vi "moveby_single_channel.vi"(4 "Desired Position":dbl) -> (1 "Sensor Sampling":waveform(dbl)[](graph), 2 "Absolute vs. Desired Pos.":cluster{dbl, "Position":dbl}(graph) caption="Waveform Chart")   [LabVIEW 2020]
uses:
  C:/Users/359167/Documents/LabVIEW_ws/Thorlabs.MotionControl.DeviceManagerCLI.dll
  Thorlabs.MotionControl.DeviceManagerCLI.dll
  C:/Users/359167/Documents/LabVIEW_ws/Thorlabs.MotionControl.KCube.InertialMotorCLI.dll
  Thorlabs.MotionControl.KCube.InertialMotorCLI.dll
  <vilib>/DAQmx/read.llb/DAQmx Read (Analog 1D Wfm NChan NSamp).vi
  <vilib>/Analysis/baseanly.llb/Mean (DBL).vi
  <vilib>/DAQmx/create/channels.llb/DAQmx Create Channel (AI-Voltage-Basic).vi
  <vilib>/DAQmx/configure/timing.llb/DAQmx Timing (Sample Clock).vi
  <vilib>/Utility/file.llb/Read Delimited Spreadsheet (DBL).vi
  <vilib>/DAQmx/miscellaneous.llb/DAQmx Fill In Error Info.vi
  <vilib>/Utility/file.llb/Write Delimited Spreadsheet (DBL).vi
  <vilib>/Analysis/NI_AALBase.lvlib
panel:
  in  "Path 2":path=path "C:/Users/359167/Documents/saved.csv"
  in  "Path":path=path "C:/Users/359167/Documents/saved.csv"
  out "Saved File Data":dbl[][](array[numeric])
  out "Absolute Pos.":dbl
  out "degree error":dbl format="%#.3f"
  out "Step Size":i32
  out "Relative Pos.":dbl
  # "Channel"
  # "Saved Abs. Pos."
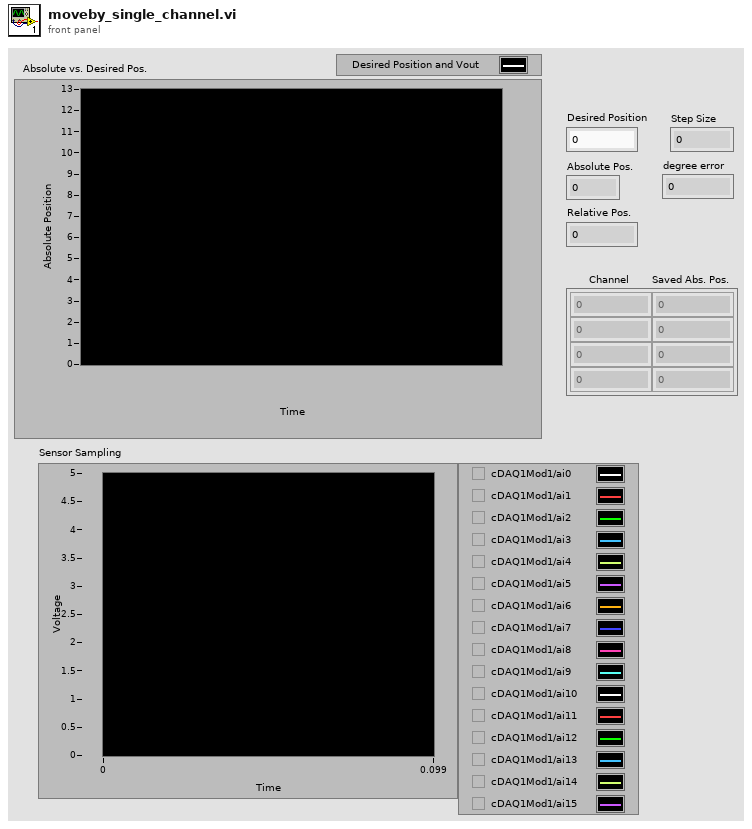
[diagram p1: front panel]
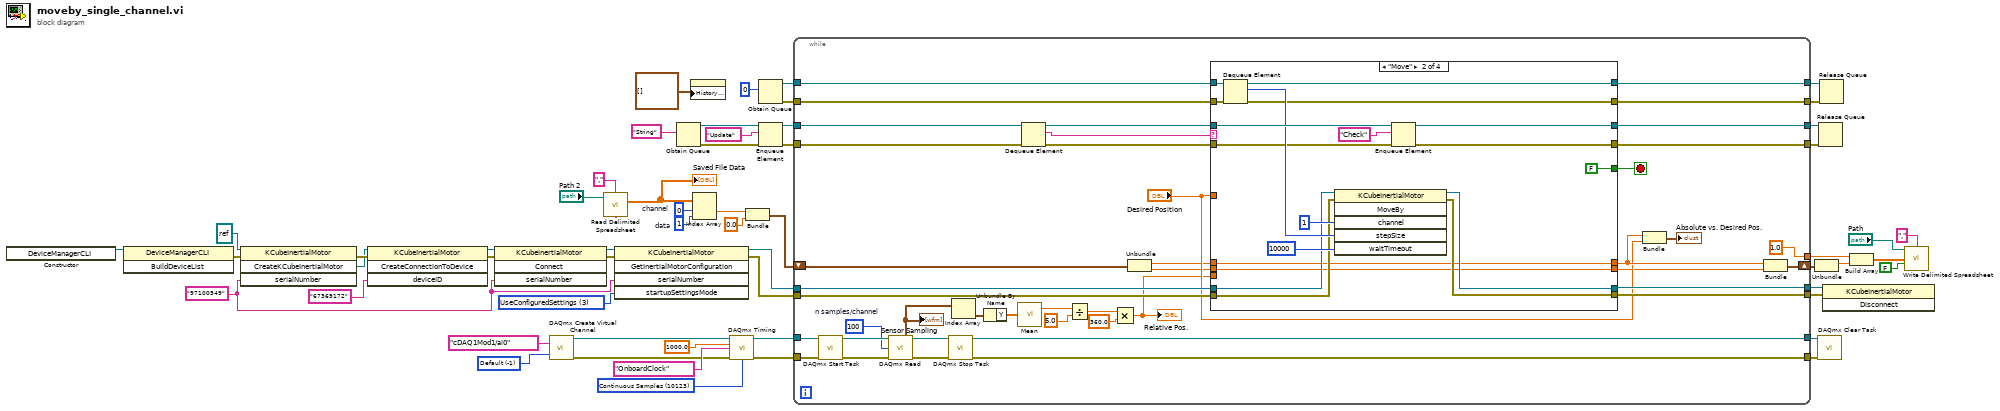
[diagram p0: block diagram]
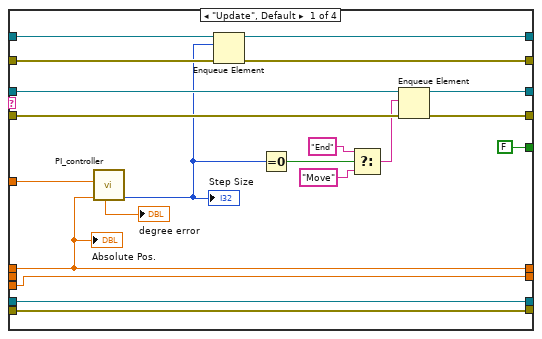
[diagram p2: hidden frame]
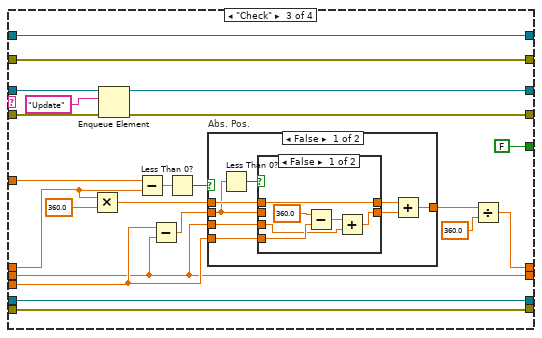
[diagram p3: hidden frame]
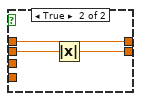
[diagram p4: hidden frame]
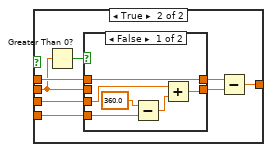
[diagram p5: hidden frame]
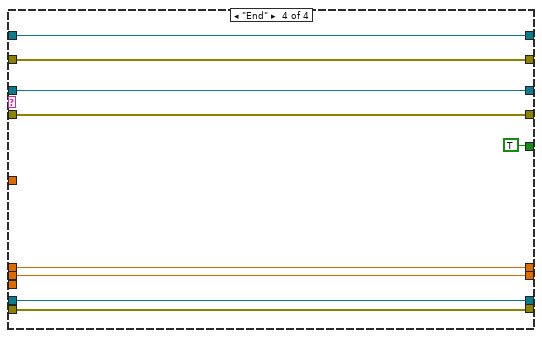
[diagram p7: hidden frame]
diagram:
  w8 = 3 items=["UseDeviceSettings"=1, "UseFileSettings"=2, "UseConfiguredSettings"=3] ("startupSettingsMode")
  w13 = "97100549" ("SerialNumber")
  w34 = -1 items=["Default"=-1, "RSE"=10083, "NRSE"=10078, "Differential"=10106, "Pseudodifferential"=12529] ("input terminal configuration")
  w35 = 10123 items=["Finite Samples"=10178, "Continuous Samples"=10123, "Hardware Timed Single Point"=12522] ("sample mode")
  w36 = 1  # data
  w37 = 0  # channel
  n1 = constructor class="DeviceManagerCLI"() -> (reference out=w26:refnum<k24>)  [unwired: 3 in, 2 out]
  n2 = invoke class="DeviceManagerCLI" method="BuildDeviceList"(reference=w26) -> (error out=w24:errorcluster)  [unwired: 2 in, 2 out]
  n3 = invoke class="KCubeInertialMotor" method="CreateKCubeInertialMotor"(reference=refnum<k24> refnum, error in=w24, "serialNumber"=w13) -> (error out=w23:errorcluster, "CreateKCubeInertialMotor"=w22:refnum<k24>)  [unwired: 1 in, 2 out]
  n4 = invoke class="KCubeInertialMotor" method="CreateConnectionToDevice"(reference=w22, error in=w23, "deviceID"="67369172") -> (reference out=w10:refnum<k24>, error out=w9:errorcluster)  [unwired: 1 in, 2 out]
  n5 = invoke class="KCubeInertialMotor" method="Connect"(reference=w10, error in=w9, "serialNumber"=w13) -> (reference out=w12:refnum<k24>, error out=w11:errorcluster)  [unwired: 1 in, 2 out]
  n6 = call-poly <vilib>:"DAQmx Create Virtual Channel.vi"("input terminal configuration"=w34, "physical channels"=tag "cDAQ1Mod1/ai0" ("DAQmx Physical Channel")) -> ("task out"=w30:refnum<k21>, "error out"=w31:errorcluster)  [unwired: 12 in]
  n7 = call-poly <vilib>:"Read Delimited Spreadsheet.vi"("file path (dialog if empty)"="Path 2", "delimiter (\\t)"="," ("delimiter (\\t)")) -> ("all rows"=w38:dbl[][])  [unwired: 8 in, 5 out]
  "Saved File Data" <- w38
  n8 = invoke class="KCubeInertialMotor" method="GetInertialMotorConfiguration"(reference=w12, error in=w11, "serialNumber"=w13, "startupSettingsMode"=w8) -> (reference out=w7:refnum<k24>, error out=w6:errorcluster)  [unwired: 1 in, 3 out]
  n9 = Obtain Queue(element data type="String") -> (queue out=w43:refnum<queue>, error out=w42:errorcluster)  [unwired: 4 in, 1 out]
  n10 = property on="Absolute vs. Desired Pos." class="WFChart (strict)"("History Data"=cluster{dbl, "Position":dbl}[] []) -> ()  [unwired: 2 in, 2 out]
  n11 = Index Array(array=w38, index (row)=w37, index (col)=w36) -> (element=w3:dbl)
  n12 = call-poly <vilib>:"DAQmx Timing.vi"("task/channels in"=w30, "sample mode"=w35, "rate"=1000.0 ("sample rate"), "source"=tag "OnboardClock", "error in"=w31) -> ("task out"=w29:refnum<k21>, "error out"=w28:errorcluster)  [unwired: 9 in]
  n13 = Bundle("Numeric"=w3, 0.0) -> (w2:cluster{"Numeric":dbl, dbl})  [unwired: 1 in]
  n14 = Obtain Queue(element data type=0) -> (queue out=w50:refnum<queue>, error out=w49:errorcluster)  [unwired: 4 in, 1 out]
  n15 = Enqueue Element(queue=w43, element="Update", error in (no error)=w42) -> (queue out=w41:refnum<queue>, error out=w40:errorcluster)  [unwired: 1 in, 1 out]
  n16 = while {
    tunnel: w50 -> [w86]
    tunnel: [w89] -> w52
    tunnel: [w90] -> w51
    tunnel: w49 -> [w88]
    tunnel: w40 -> [w71]
    tunnel: [w87] -> w48
    tunnel: [w74] -> w47
    tunnel: [w68] -> w46
    tunnel: [w67] -> w45
    tunnel: w41 -> [w72]
    tunnel: [1.0] -> w18
    tunnel: w7 -> [w65]
    tunnel: w6 -> [w64]
    tunnel: w29 -> [w94]
    tunnel: [w92] -> w56
    tunnel: w28 -> [w93]
    tunnel: [w91] -> w55
    shift-right: [w66] -> w5
    shift-left: w2 -> [w60]
    stop <- w96 stop-if-true
    w81 = 100  # n samples/channel
    # "Consumer"
    n17 = call <vilib>:"DAQmx Start Task.vi"("task/channels in"=w94, "error in"=w93) -> ("task out"=w82:refnum<k21>, "error out"=w83:errorcluster)  [unwired: 12 in]
    n18 = call-poly <vilib>:"DAQmx Read.vi"("task/channels in"=w82, "number of samples per channel"=w81, "error in"=w83) -> ("data"=w70:waveform(dbl)[], "task out"=w84:refnum<k21>, "error out"=w85:errorcluster)  [unwired: 10 in]
    "Sensor Sampling" <- w70
    n19 = call <vilib>:"DAQmx Stop Task.vi"("task/channels in"=w84, "error in"=w85) -> ("task out"=w92:refnum<k21>, "error out"=w91:errorcluster)  [unwired: 12 in]
    n20 = Index Array(array=w70) -> (element=w80:waveform(dbl))  [unwired: 1 in]
    n21 = Unbundle By Name(w80) -> ("Y"=w78:dbl[])
    n22 = call-poly <vilib>:"Mean.vi"("X"=w78) -> ("mean"=w77:dbl)  [unwired: 1 out]
    n23 = Dequeue Element(queue=w72, error in (no error)=w71) -> (queue out=w98:refnum<queue>, element=w97:string, error out=w95:errorcluster)  [unwired: 1 in, 1 out]
    n24 = Divide(x=w77, y=5.0) -> (x/y=w79:dbl)
    n25 = Multiply(x=w79, y=360.0) -> (x*y=w61:dbl)
    "Relative Pos." <- w61
    n26 = Unbundle(w60) -> ("Numeric"=w57:dbl, w58:dbl)
    n27 = case shown="\"Move\"" w97 {
      tunnel: w98 -> [w112 w135 w156 w198]
      tunnel: [w118 w125 w157 w199] -> w87
      tunnel: [FALSE FALSE FALSE TRUE] -> w96
      tunnel: w95 -> [w117 w132 w155 w199]
      tunnel: w86 -> [w116 w129 w154 w200]
      tunnel: w88 -> [w115 w131 w153 w197]
      tunnel: [w114 w128 w154 w200] -> w74
      tunnel: [w113 w130 w153 w197] -> w68
      tunnel: [w102 w137 w142 w195] -> w90
      tunnel: [w103 w136 w143 w196] -> w89
      tunnel: [w108 w127 w158 w198] -> w67
      tunnel: [w100 w120 w148 w194] -> w63
      tunnel: [w99 w119 w138 w193] -> w59
      tunnel: w65 -> [w102 w122 w142 w195]
      tunnel: w64 -> [w103 w121 w143 w196]
      tunnel: "Desired Position" -> [w101 _ w141 _]
      tunnel: w61 -> [w99 _ w140 _]
      tunnel: w57 -> [w100 w120 w139 w194]
      tunnel: w58 -> [_ w119 w138 w193]
      frame "Update", Default {
        n28 = call "PI_controller.vi"("absolute position"=w100, "desired position"=w101) -> ("step size"=w107:i32, "degree error"=→"degree error":dbl)  [unwired: 7 in, 1 out]
        "Step Size" <- w107
        n29 = Enqueue Element(queue=w116, element=w107, error in (no error)=w115) -> (queue out=w114:refnum<queue>, error out=w113:errorcluster)  [unwired: 1 in, 1 out]
        n30 = Equal To 0?(x=w107) -> (x = 0?=w105:bool)
        n31 = Select(t="End", s=w105, f="Move" ("element")) -> (s? t:f=w109:string)
        n32 = Enqueue Element(queue=w112, element=w109, error in (no error)=w117) -> (queue out=w108:refnum<queue>, error out=w118:errorcluster)  [unwired: 1 in, 1 out]
        "Absolute Pos." <- w100
      }
      frame "Move" {
        n33 = Dequeue Element(queue=w129, error in (no error)=w131) -> (queue out=w128:refnum<queue>, element=w134:i32, error out=w130:errorcluster)  [unwired: 1 in, 1 out]
        n34 = invoke class="KCubeInertialMotor" method="MoveBy"(reference=w122, error in=w121, "channel"=1 ("Channel"), "stepSize"=w134, "waitTimeout"=10000) -> (reference out=w137:refnum<k24>, error out=w136:errorcluster)  [unwired: 1 in, 4 out]
        n35 = Enqueue Element(queue=w135, element="Check", error in (no error)=w132) -> (queue out=w127:refnum<queue>, error out=w125:errorcluster)  [unwired: 1 in, 1 out]
      }
      frame "Check" {
        n36 = Multiply(x=w139, y=360.0) -> (x*y=w144:dbl)
        n37 = Enqueue Element(queue=w156, element="Update", error in (no error)=w155) -> (queue out=w158:refnum<queue>, error out=w157:errorcluster)  [unwired: 1 in, 1 out]
        n38 = Subtract(x=w141, y=w139) -> (x-y=w147:dbl)
        n39 = Subtract(x=w140, y=w138) -> (x-y=w146:dbl)
        n40 = Less Than 0?(x=w147) -> (x < 0?=w151:bool)
        n41 = case "Abs. Pos." shown="False" w151 {
          tunnel: w144 -> [w164 w184]
          tunnel: w138 -> [w166 w182]
          tunnel: [w165 w180] -> w150
          tunnel: w140 -> [w161 w178]
          tunnel: w146 -> [w160 w177]
          frame False {
            n42 = Less Than 0?(x=w160) -> (x < 0?=w167:bool)
            n43 = case shown="False" w167 {
              tunnel: w164 -> [w171 w176]
              tunnel: [w172 w174] -> w162
              tunnel: w166 -> [w168 _]
              tunnel: w161 -> [w169 _]
              tunnel: [w171 w176] -> w163
              tunnel: w160 -> [_ w175]
              frame False {
                n44 = Subtract(x=360.0 ("y"), y=w169) -> (x-y=w173:dbl)
                n45 = Add(x=w173, y=w168) -> (x+y=w172:dbl)
              }
              frame True {
                n46 = Absolute Value(x=w175) -> (abs(x)=w174:dbl)
              }
            }
            n47 = Add(x=w163, y=w162) -> (x+y=w165:dbl)
          }
          frame True {
            n48 = Greater Than 0?(x=w177) -> (x > 0?=w183:bool)
            n49 = case shown="False" w183 {
              tunnel: w184 -> [w187 w192]
              tunnel: w177 -> [_ w191]
              tunnel: w182 -> [w190 _]
              tunnel: [w188 w191] -> w181
              tunnel: [w187 w192] -> w179
              tunnel: w178 -> [w185 _]
              frame False {
                n50 = Subtract(x=360.0, y=w185) -> (x-y=w189:dbl)
                n51 = Add(x=w190, y=w189) -> (x+y=w188:dbl)
              }
              frame True {
              }
            }
            n52 = Subtract(x=w179, y=w181) -> (x-y=w180:dbl)
          }
        }
        n53 = Divide ("absolute position")(x=w150, y=360.0) -> (x/y=w148:dbl)
      }
      frame "End" {
      }
    }
    n54 = Bundle("Numeric"=w63, "Desired Position"="Desired Position") -> (→"Absolute vs. Desired Pos.":cluster{"Numeric":dbl, "Desired Position":dbl})  [unwired: 1 in]
    n55 = Bundle("Numeric"=w63, w59) -> (w66:cluster{"Numeric":dbl, dbl})  [unwired: 1 in]
  }
  n56 = Unbundle(w5) -> ("Numeric"=w4:dbl)  [unwired: 1 out]
  n57 = call <vilib>:"DAQmx Clear Task.vi"("task in"=w56, "error in"=w55) -> ()  [unwired: 13 in, 1 out]
  n58 = Release Queue(queue=w45, error in (no error)=w48) -> ()  [unwired: 1 in, 3 out]
  n59 = Release Queue(queue=w47, error in (no error)=w46) -> ()  [unwired: 1 in, 3 out]
  n60 = invoke class="KCubeInertialMotor" method="Disconnect"(reference=w51, error in=w52) -> ()  [unwired: 1 in, 3 out]
  n61 = Build Array(w18, w4) -> (w17:dbl[])
  n62 = call-poly <vilib>:"Write Delimited Spreadsheet.vi"("file path (dialog if empty)"="Path", "1D data"=w17, "append to file? (new file:F)"=FALSE, "delimiter (\\t)"="," ("delimiter (\\t)")) -> ()  [unwired: 10 in, 2 out]
